vi "Generate RID.vi"(10 "Negative? (F)":bool, 11 "LUT in":variant) -> (2 "Unique Key":string, 3 "LUT out":variant)   [LabVIEW 2013, in "SET Project Data.lvlib"]
uses:
  SET Project Data.lvlib
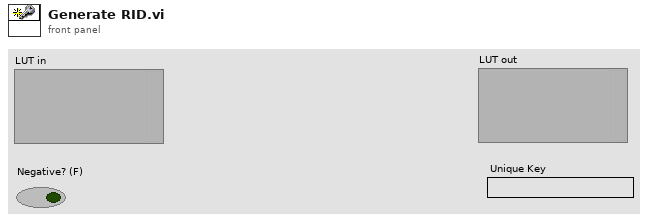
[diagram p1: front panel]
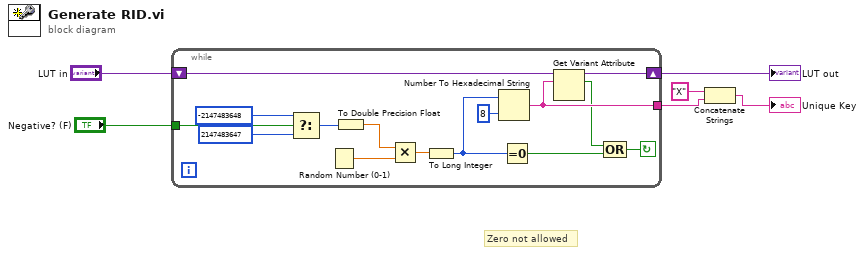
[diagram p0: block diagram]
diagram:
  # "Zero not allowed"
  n1 = while {
    tunnel: "Negative? (F)" -> [w16]
    shift-right: [w12] -> w5
    shift-left: "LUT in" -> [w18]
    tunnel: [w11] -> w2
    stop <- w7 continue-if-true
    n2 = Select(t=-2147483648, s=w16, f=2147483647) -> (s? t:f=w14:i32)
    n3 = Random Number (0-1)() -> (number: 0 to 1=w20:dbl)
    n4 = To Double Precision Float(number=w14) -> (double precision float=w21:dbl)
    n5 = Multiply(x=w21, y=w20) -> (x*y=w19:dbl)
    n6 = To Long Integer(number=w19) -> (32bit integer=w10:i32)
    n7 = Number To Hexadecimal String(1:i16 8 ("width (-)"), 2:w10) -> (0:w11:string)
    n8 = Equal To 0?(x=w10) -> (x = 0?=w9:bool)
    n9 = Get Variant Attribute(Variant=w18, name=w11) -> (duplicate Variant=w12:variant, found=w8:bool)  [unwired: 2 in, 2 out]
    n10 = Compound Arithmetic op=OR(w8, w9) -> (w7:bool)
  }
  "LUT out" <- w5
  n11 = Concatenate Strings("X", w2) -> (→"Unique Key":string)
